vi "A_6.vi"() -> ()   [LabVIEW 2020]
panel:
  out "Time in sec":dbl
  out "Second number":dbl
  out "First number":dbl
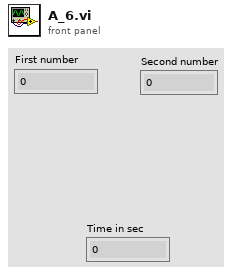
[diagram p1: front panel]
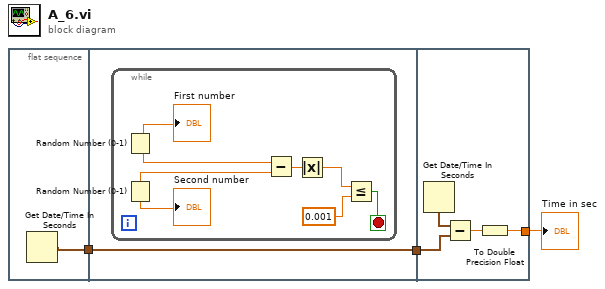
[diagram p0: block diagram]
diagram:
  n1 = flat-sequence {
    tunnel: [w4] -> w2
    tunnel: [w5] -> w3
    tunnel: w2 -> [w5]
    tunnel: w3 -> [w15]
    tunnel: [w13] -> w1
    frame #0 {
      n2 = Get Date/Time In Seconds() -> (seconds since 1Jan1904=w4:timestamp)
    }
    frame #1 {
      n3 = while {
        stop <- w8 stop-if-true
        n4 = Random Number (0-1)() -> (number: 0 to 1=w7:dbl)
        "First number" <- w7
        n5 = Random Number (0-1)() -> (number: 0 to 1=w6:dbl)
        "Second number" <- w6
        n6 = Subtract(x=w7, y=w6) -> (x-y=w11:dbl)
        n7 = Absolute Value(x=w11) -> (abs(x)=w10:dbl)
        n8 = Less Or Equal?(x=w10, y=0.001) -> (x <= y?=w8:bool)
      }
    }
    frame #2 {
      n9 = Get Date/Time In Seconds() -> (seconds since 1Jan1904=w12:timestamp)
      n10 = Subtract(x=w12, y=w15) -> (x-y=w14:dbl)
      n11 = To Double Precision Float(number=w14) -> (double precision float=w13:dbl)
    }
  }
  "Time in sec" <- w1
